vi "Calculate Shooter Speed.vi"(11 "Shoot":bool) -> (3 "Shooter Speed out":dbl)   [LabVIEW 2020]
uses:
  Robot Global Data.vi
  <vilib>/Rock Robotics/Network Tables/NT Read Numeric Array.vi
  2017 Swerve Code/Swerve Global Variables.vi
panel:
  in  "speed lookup table":dbl[](array[numeric])
  out "Raspberry pi info":dbl[](array[numeric])
  in  "Default Shooter Speed in":dbl=3100.0
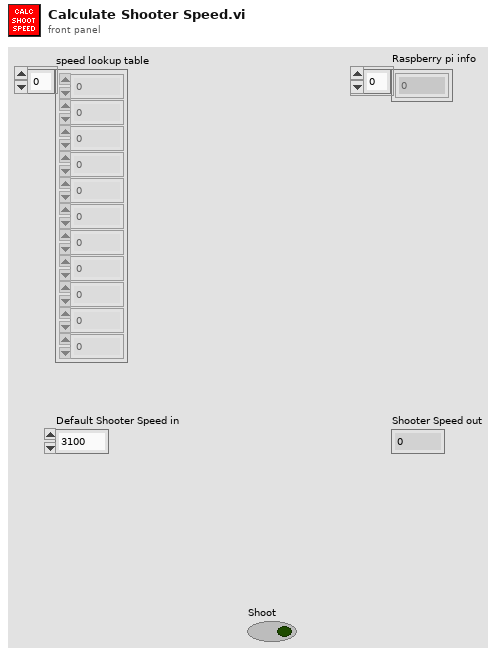
[diagram p1: front panel]
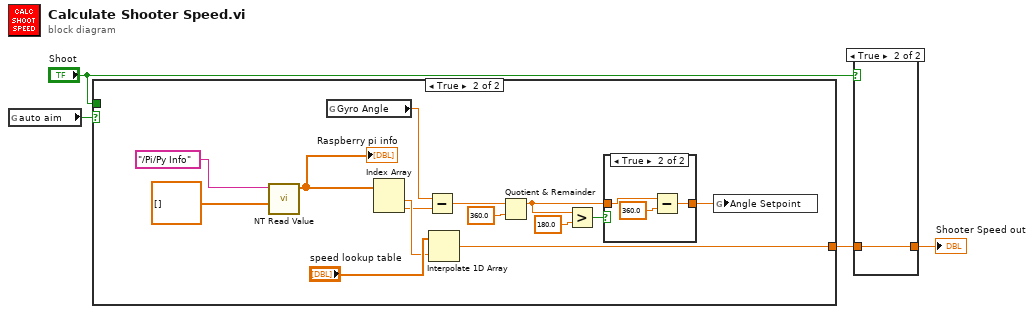
[diagram p0: block diagram]
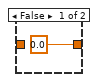
[diagram p2: hidden frame]
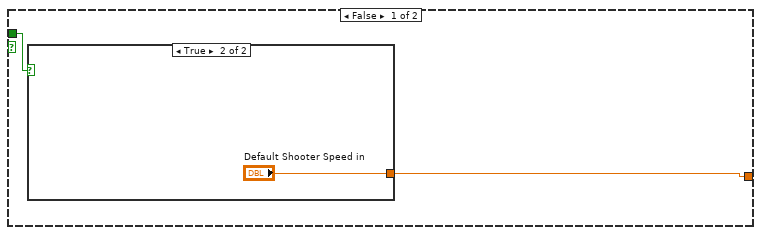
[diagram p3: hidden frame]
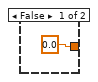
[diagram p4: hidden frame]
diagram:
  n1 = global read "Robot Global Data.vi" "auto aim"() -> (w1:bool)
  n2 = case shown="True" w1 {
    tunnel: [w5 w17] -> w2
    tunnel: "Shoot" -> [w6 _]
    frame False {
      n3 = case shown="True" w6 {
        tunnel: [0.0 "Default Shooter Speed in"] -> w5
        frame False {
        }
        frame True {
        }
      }
    }
    frame True {
      n4 = call-poly <vilib>:"NT Read Value.vi"("Default Value"=dbl[] [], "Name"="/Pi/Py Info") -> ("Numeric Array"=w20:dbl[])  [unwired: 8 in, 1 out]
      "Raspberry pi info" <- w20
      n5 = global read "Swerve Global Variables.vi" "Gyro Angle"() -> (w16:dbl)
      n6 = Index Array(array=w20) -> (element #1=w18:dbl, element #2=w9:dbl)  [unwired: 2 in]
      n7 = Subtract(x=w16, y=w9) -> (x-y=w15:dbl)
      n8 = Interpolate 1D Array(1:w18, 2:"speed lookup table") -> (0:w17:dbl)
      n9 = Quotient & Remainder(x=w15, y=360.0) -> (x-y*floor(x/y)=w11:dbl)  [unwired: 1 out]
      n10 = Greater?(x=w11, y=180.0) -> (0:w12:bool)
      n11 = case shown="True" w12 {
        tunnel: [w23 w24] -> w10
        tunnel: w11 -> [w23 w26]
        frame False {
        }
        frame True {
          n12 = Subtract(x=w26, y=360.0) -> (x-y=w24:dbl)
        }
      }
      n13 = global write "Robot Global Data.vi" "Angle Setpoint"(w10) -> ()
    }
  }
  n14 = case shown="True" "Shoot" {
    tunnel: [0.0 w28] -> w3
    tunnel: w2 -> [_ w28]
    frame False {
    }
    frame True {
    }
  }
  "Shooter Speed out" <- w3
